vi "_markSFP+&QSFP+_EEPROM_vna_wmg.vi"(0 "枚举":enum16{"0", "1"}(ring), 1 "chart_step2 2":refnum<vi>) -> ()   [LabVIEW 2011]
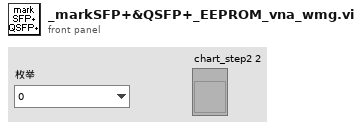
[diagram p1: front panel]
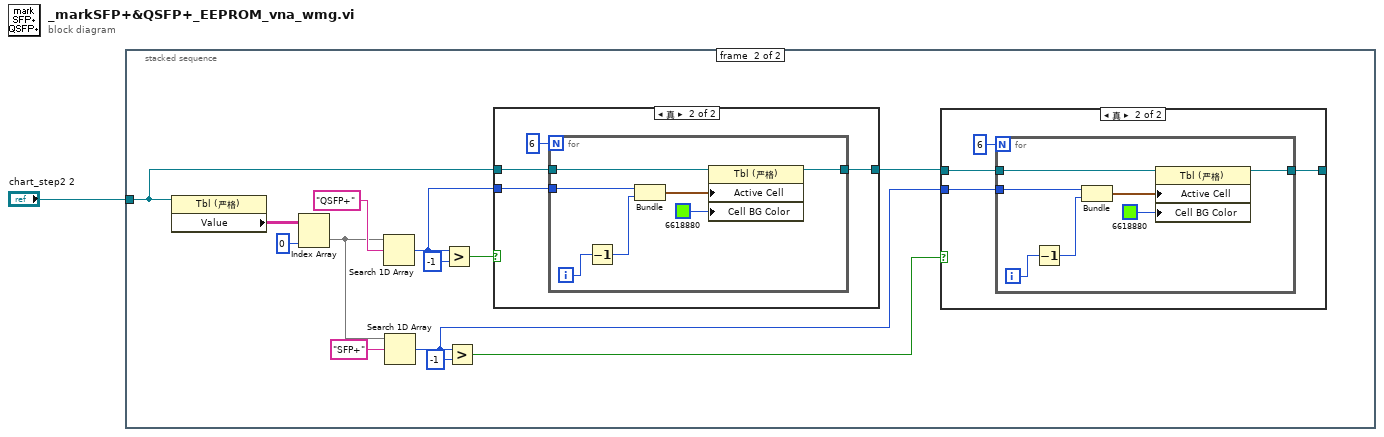
[diagram p0: block diagram]
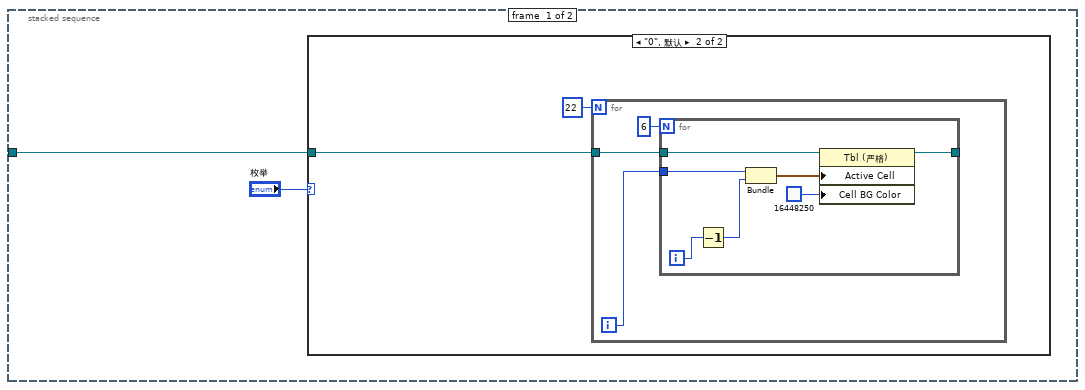
[diagram p2: hidden frame]
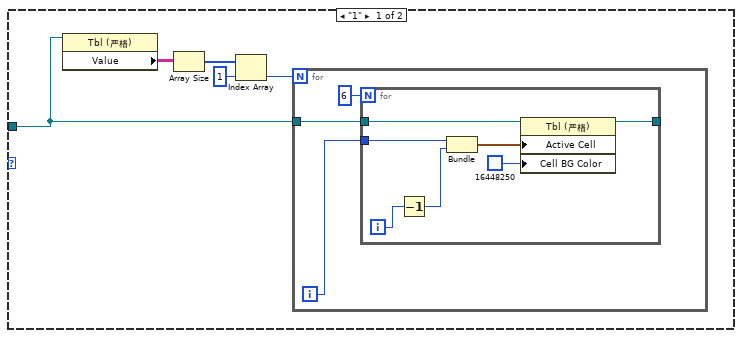
[diagram p3: hidden frame]
diagram:
  n1 = stacked-sequence {
    tunnel: "chart_step2 2" -> [w3 w35]
    frame #0 {
      n2 = case shown="\"0\", 默认" "枚举" {
        tunnel: w3 -> [w4 w20]
        frame "1" {
          n3 = property class="Tbl (严格)"(reference=w4) -> ("Value"=w8:string[][])  [unwired: 1 in, 2 out]
          n4 = Array Size(array=w8) -> (size(s)=w7:i32[])
          n5 = Index Array(array=w7, index=1 ("索引")) -> (element=w5:i32)
          n6 = for {
            N: w5 -> [_]
            tunnel: w4 -> [w10]
            i -> [w9]
            n7 = for {
              N: 6 -> [_]
              tunnel: w10 -> [w18]
              tunnel: w9 -> [w16]
              tunnel: [w12] -> _
              i -> [w17]
              n8 = Decrement(x=w17) -> (x-1=w15:i32)
              n9 = Bundle(w16, w15) -> (w14:cluster{i32, i32})  [unwired: 1 in]
              n10 = property class="Tbl (严格)"(reference=w18, "Active Cell"=w14, "Cell BG Color"=u32 16448250) -> (reference out=w12:refnum<vi>)  [unwired: 1 in, 1 out]
            }
          }
        }
        frame "0", Default {
          n11 = for {
            N: 22 -> [_]
            tunnel: w20 -> [w22]
            i -> [w21]
            n12 = for {
              N: 6 -> [_]
              tunnel: w22 -> [w30]
              tunnel: w21 -> [w28]
              tunnel: [w24] -> _
              i -> [w29]
              n13 = Decrement(x=w29) -> (x-1=w27:i32)
              n14 = Bundle(w28, w27) -> (w26:cluster{i32, i32})  [unwired: 1 in]
              n15 = property class="Tbl (严格)"(reference=w30, "Active Cell"=w26, "Cell BG Color"=u32 16448250) -> (reference out=w24:refnum<vi>)  [unwired: 1 in, 1 out]
            }
          }
        }
      }
    }
    frame #1 {
      n16 = property class="Tbl (严格)"(reference=w35) -> ("Value"=w43:string[][])  [unwired: 1 in, 2 out]
      n17 = Index Array(array=w43, index (col)=0 ("禁用的索引 (列)")) -> (element=w40:string[])  [unwired: 1 in]
      n18 = Search 1D Array(1D array=w40, element="QSFP+" ("元素")) -> (index of element=w34:i32)  [unwired: 1 in]
      n19 = Search 1D Array(1D array=w40, element="SFP+" ("元素")) -> (index of element=w32:i32)  [unwired: 1 in]
      n20 = Greater?(x=w34, y=-1) -> (0:w36:bool)
      n21 = Greater?(x=w32, y=-1) -> (0:w31:bool)
      n22 = case shown="真" w36 {
        tunnel: w35 -> [w56 w60]
        tunnel: w34 -> [_ w58]
        tunnel: [w56 w57] -> w33
        frame False {
        }
        frame True {
          n23 = for {
            N: 6 -> [_]
            tunnel: w60 -> [w67]
            tunnel: w58 -> [w65]
            tunnel: [w61] -> w57
            i -> [w66]
            n24 = Decrement(x=w66) -> (x-1=w64:i32)
            n25 = Bundle("index of element"=w65, w64) -> (w63:cluster{"index of element":i32, i32})  [unwired: 1 in]
            n26 = property class="Tbl (严格)"(reference=w67, "Active Cell"=w63, "Cell BG Color"=u32 6618880) -> (reference out=w61:refnum<vi>)  [unwired: 1 in, 1 out]
          }
        }
      }
      n27 = case shown="真" w31 {
        tunnel: w33 -> [w44 w48]
        tunnel: [w44 w46] -> _
        tunnel: w32 -> [_ w45]
        frame False {
        }
        frame True {
          n28 = for {
            N: 6 -> [_]
            tunnel: w48 -> [w55]
            tunnel: w45 -> [w53]
            tunnel: [w49] -> w46
            i -> [w54]
            n29 = Decrement(x=w54) -> (x-1=w52:i32)
            n30 = Bundle("index of element"=w53, w52) -> (w51:cluster{"index of element":i32, i32})  [unwired: 1 in]
            n31 = property class="Tbl (严格)"(reference=w55, "Active Cell"=w51, "Cell BG Color"=u32 6618880) -> (reference out=w49:refnum<vi>)  [unwired: 1 in, 1 out]
          }
        }
      }
    }
  }
